vi "XML Parsing.vi"(8 "error in (no error)":errorcluster, 10 "File Type":enum16{"XML", "RML"}(ring), 11 "XML File Path":path) -> (0 "error out":errorcluster, 2 "Offset Time":string[](array[string]), 3 "XML Notes and Times":string[][](array[string]))   [LabVIEW 2021]
uses:
  <vilib>/xml/Close Reference(Node).vi
  <vilib>/xml/NI_XML.lvlib
  <resource>/objmgr/DOMUserDefRef.rc
panel:
  out "XML":string
  out "Parse Errors":string
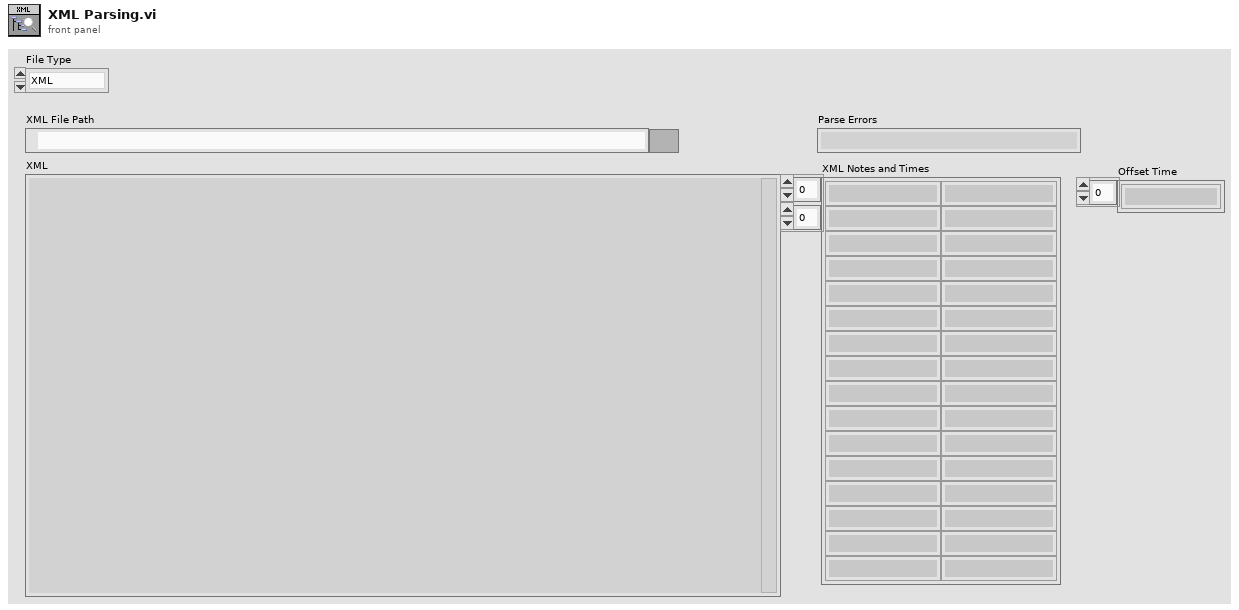
[diagram p1: front panel]
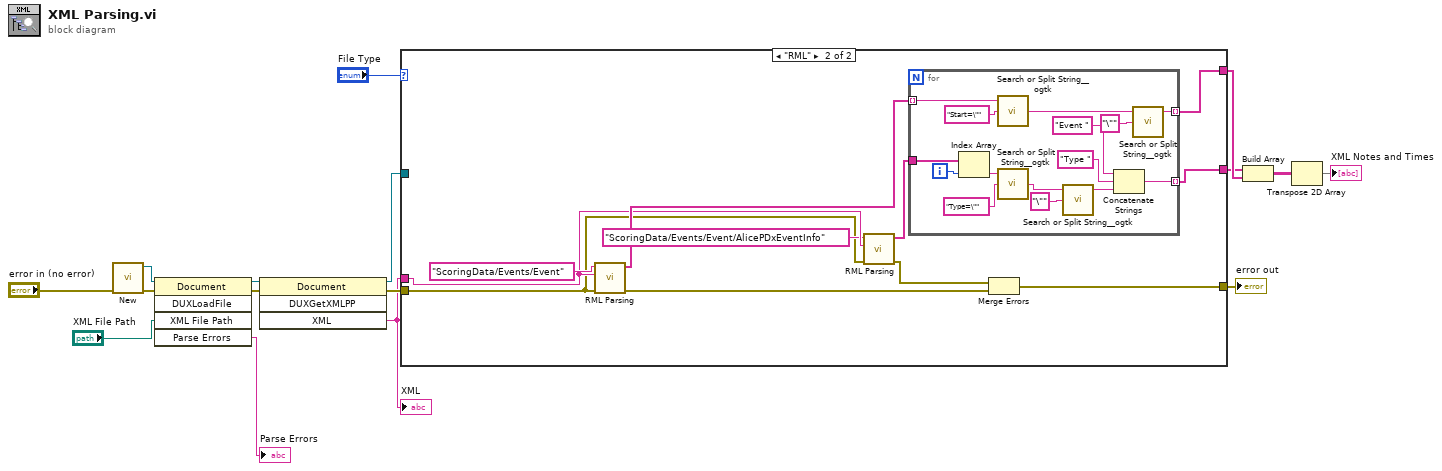
[diagram p0: block diagram]
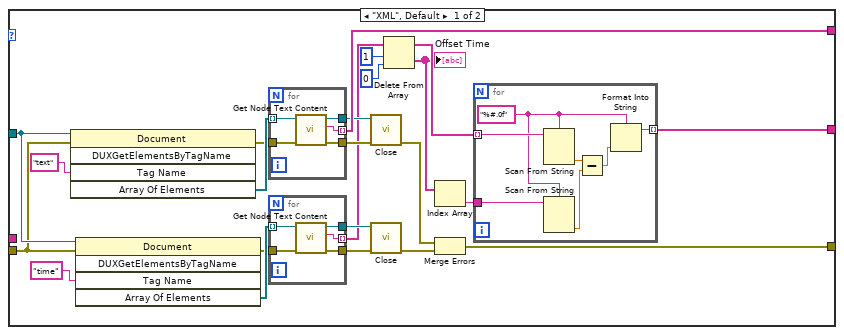
[diagram p2: hidden frame]
diagram:
  n1 = call <vilib>:"New.vi"("error in (no error)"="error in (no error)") -> ("error out"=w15:errorcluster, "DOM document out"=w16:refnum<k20>)  [unwired: 7 in]
  n2 = invoke class="Document" method="DUXLoadFile"(reference=w16, error in=w15, "XML File Path"="XML File Path") -> (reference out=w13:refnum<k20>, error out=w12:errorcluster, "Parse Errors"=→"Parse Errors":string)  [unwired: 2 in, 2 out]
  n3 = invoke class="Document" method="DUXGetXMLPP"(reference=w13, error in=w12) -> (reference out=w6:refnum<k20>, error out=w5:errorcluster, "XML"=w1:string)  [unwired: 2 in, 1 out]
  "XML" <- w1
  n4 = case shown="\"RML\"" "File Type" {
    tunnel: w6 -> [w38 _]
    tunnel: w5 -> [w37 w60]
    tunnel: [w32 w65] -> w4
    tunnel: [w24 w57] -> w3
    tunnel: [w17 w64] -> w2
    tunnel: w1 -> [_ w63]
    frame "XML", Default {
      n5 = invoke class="Document" method="DUXGetElementsByTagName"(reference=w38, error in=w37, "Tag Name"="text") -> (error out=w33:errorcluster, "Array Of Elements"=w34:refnum<k20>[])  [unwired: 2 in, 3 out]
      n6 = invoke class="Document" method="DUXGetElementsByTagName"(reference=w38, error in=w37, "Tag Name"="time") -> (error out=w31:errorcluster, "Array Of Elements"=w35:refnum<k20>[])  [unwired: 2 in, 3 out]
      n7 = for {
        tunnel: w34 -> [w56] mode=indexing
        tunnel: [w55] -> w32 mode=indexing
        tunnel: w33 -> [w54]
        tunnel: [w53] -> w28
        tunnel: [w52] -> w27
        n8 = call <vilib>:"Get Node Text Content.vi"("error in (no error)"=w54, "node in"=w56) -> ("error out"=w53:errorcluster, "node text"=w55:string, "node out"=w52:refnum<k20>)  [unwired: 7 in]
      }
      n9 = for {
        tunnel: [w51] -> w20 mode=indexing
        tunnel: [w50] -> w30
        tunnel: [w49] -> w29
        tunnel: w35 -> [w48] mode=indexing
        tunnel: w31 -> [w47]
        n10 = call <vilib>:"Get Node Text Content.vi"("error in (no error)"=w47, "node in"=w48) -> ("error out"=w50:errorcluster, "node text"=w51:string, "node out"=w49:refnum<k20>)  [unwired: 7 in]
      }
      n11 = call-poly <vilib>:"Close.vi"("error in (no error)"=w28, "node"=w27) -> ("error out"=w26:errorcluster)  [unwired: 7 in]
      n12 = call-poly <vilib>:"Close.vi"("error in (no error)"=w30, "node"=w29) -> ("error out"=w25:errorcluster)  [unwired: 7 in]
      n13 = Delete From Array(array=w20, length=1, index=0) -> (deleted portion=w21:string[], array with subset deleted=w23:string[])
      "Offset Time" <- w21
      n14 = Index Array(array=w21) -> (element=w22:string)  [unwired: 1 in]
      n15 = Merge Errors(w26, w25) -> (w24:errorcluster)
      n16 = for {
        tunnel: w22 -> [w45]
        tunnel: w23 -> [w46] mode=indexing
        tunnel: [w41] -> w17 mode=indexing
        w40 = "%#.0f" ("format string")
        n17 = Scan From String(format string=w40, input string=w46) -> (output 1=w44:dbl)  [unwired: 3 in, 3 out]
        n18 = Scan From String(format string=w40, input string=w45) -> (output 1=w43:dbl)  [unwired: 3 in, 3 out]
        n19 = Subtract(x=w44, y=w43) -> (x-y=w42:dbl)
        n20 = Format Into String(format string=w40, w42) -> (resulting string=w41:string)  [unwired: 2 in, 1 out]
      }
    }
    frame "RML" {
      n21 = call "RML Parsing.vi"("error in (no error)"=w60, "XML String"=w63, "XPath Expression"="ScoringData/Events/Event" ("XPath expression")) -> ("error out"=w58:errorcluster, "Search Results"=w66:string[])  [unwired: 7 in]
      n22 = call "RML Parsing.vi"("error in (no error)"=w60, "XML String"=w63, "XPath Expression"="ScoringData/Events/Event/AlicePDxEventInfo" ("XPath expression")) -> ("error out"=w59:errorcluster, "Search Results"=w61:string[])  [unwired: 7 in]
      n23 = for {
        tunnel: w66 -> [w82] mode=indexing
        tunnel: [w78] -> w65 mode=indexing
        tunnel: [w68] -> w64 mode=indexing
        tunnel: w61 -> [w77]
        i -> [w69]
        n24 = Index Array(array=w77, index=w69) -> (element=w76:string)
        n25 = call <userlib>:"Search or Split String__ogtk.vi"("search string/char (-)"="Start=\"", "string"=w82) -> ("substring after match"=w80:string)  [unwired: 1 in, 2 out]
        n26 = call <userlib>:"Search or Split String__ogtk.vi"("search string/char (-)"="Type=\"", "string"=w76) -> ("substring after match"=w74:string)  [unwired: 1 in, 2 out]
        n27 = call <userlib>:"Search or Split String__ogtk.vi"("search string/char (-)"="\"", "string"=w74) -> ("substring before match"=w70:string)  [unwired: 1 in, 2 out]
        n28 = Concatenate Strings("Event ", "Type " ("string"), w70) -> (w68:string)
        n29 = call <userlib>:"Search or Split String__ogtk.vi"("search string/char (-)"="\"", "string"=w80) -> ("substring before match"=w78:string)  [unwired: 1 in, 2 out]
      }
      n30 = Merge Errors(w59, w58) -> (w57:errorcluster)
    }
  }
  "error out" <- w3
  n31 = Build Array(w2, w4) -> (w9:string[][])
  n32 = Transpose 2D Array(2D array=w9) -> (transposed array=→"XML Notes and Times":string[][])
